vi "LED indicator (SubVI).vi"(11 "index of element":i32) -> (0 "Boolean 4":bool, 1 "Boolean 3":bool, 2 "Boolean 2":bool, 3 "Boolean":bool)   [LabVIEW 2013]
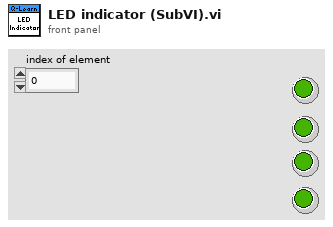
[diagram p1: front panel]
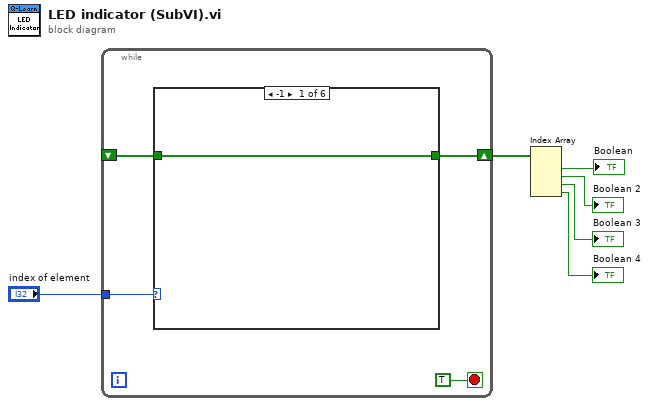
[diagram p0: block diagram]
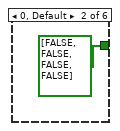
[diagram p2: hidden frame]
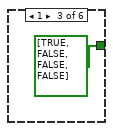
[diagram p3: hidden frame]
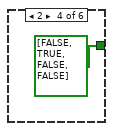
[diagram p4: hidden frame]
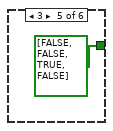
[diagram p5: hidden frame]
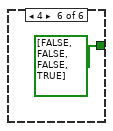
[diagram p6: hidden frame]
diagram:
  n1 = while {
    tunnel: "index of element" -> [w10]
    shift-right: [w8] -> w1
    shift-left: _ -> [w9]
    stop <- TRUE stop-if-true
    n2 = case shown="-1" w10 {
      tunnel: w9 -> [w11 _ _ _ _ _]
      tunnel: [w11 bool[] [FALSE, FALSE, FALSE, FALSE] bool[] [TRUE, FALSE, FALSE, FALSE] bool[] [FALSE, TRUE, FALSE, FALSE] bool[] [FALSE, FALSE, TRUE, FALSE] bool[] [FALSE, FALSE, FALSE, TRUE]] -> w8
      frame -1 {
      }
      frame 0, Default {
      }
      frame 1 {
      }
      frame 2 {
      }
      frame 3 {
      }
      frame 4 {
      }
    }
  }
  n3 = Index Array(array=w1) -> (element #1=→"Boolean":bool, element #2=→"Boolean 2":bool, element #3=→"Boolean 3":bool, element #4=→"Boolean 4":bool)  [unwired: 4 in]
